vi "Windspeed Warnings.vi"(8 "错误输入":cluster{"状态":bool, "代码":i32, "源":string}, 10 "最大风速":dbl, 11 "当前风速":dbl) -> (0 "错误输出":cluster{"状态":bool, "代码":i32, "源":string}, 2 "风速警告文本":string="无警告", 3 "风速警告？":bool)   [LabVIEW 2012]
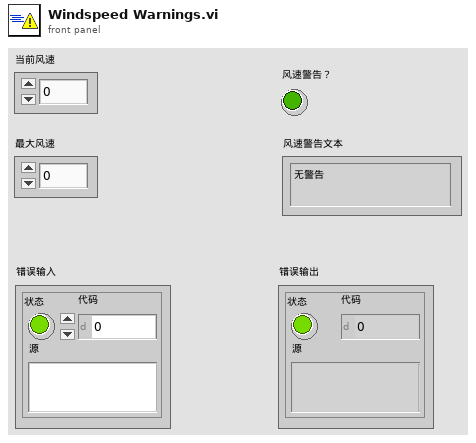
[diagram p1: front panel]
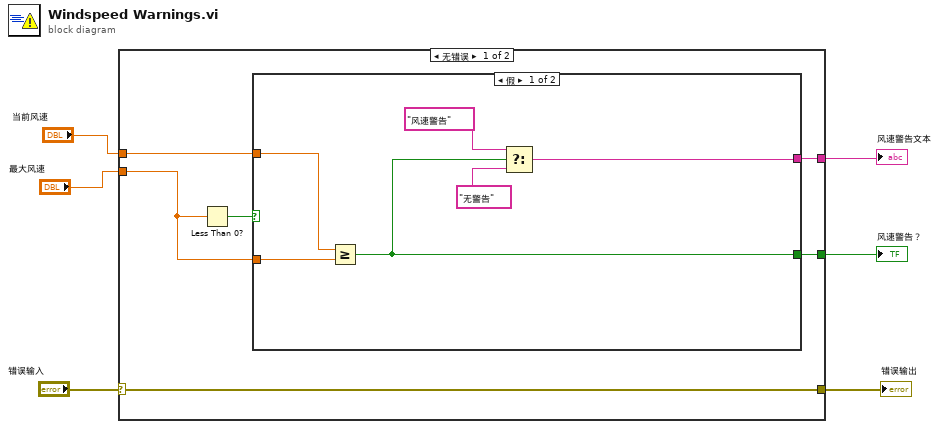
[diagram p0: block diagram]
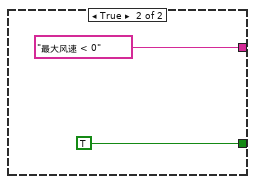
[diagram p2: hidden frame]
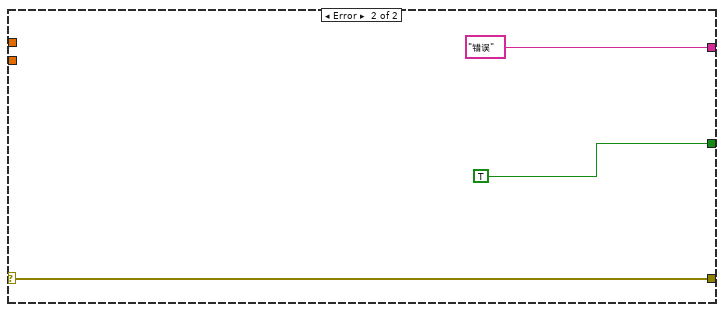
[diagram p3: hidden frame]
diagram:
  n1 = case shown="无错误" "错误输入" {
    selector: "错误输入" -> [w9 w23]
    tunnel: [w12 "错误" ("f")] -> w1
    tunnel: [w11 TRUE] -> w2
    tunnel: [w9 w23] -> w5
    tunnel: "当前风速" -> [w8 _]
    tunnel: "最大风速" -> [w7 _]
    frame No Error {
      n2 = Less Than 0? ("小于0？")(x=w7) -> (x < 0?=w10:bool)
      n3 = case shown="假" w10 {
        tunnel: [w14 "最大风速 < 0" ("f")] -> w12
        tunnel: [w13 TRUE] -> w11
        tunnel: w7 -> [w18 _]
        tunnel: w8 -> [w15 _]
        frame False {
          n4 = Greater Or Equal? ("大于等于？")(x=w15, y=w18) -> (x >= y?=w13:bool)
          n5 = Select ("选择")(t="风速警告", s=w13, f="无警告") -> (s? t:f=w14:string)
        }
        frame True {
        }
      }
    }
    frame Error {
    }
  }
  "错误输出" <- w5
  "风速警告？" <- w2
  "风速警告文本" <- w1
